vi "uv decode.vi"(8 "error in (no error)":errorcluster, 9 "para2":cluster{}, 10 "para1":cluster{}, 11 "para0":cluster{}) -> (0 "error out":errorcluster, 1 "function return":i32, 2 "para1 out":cluster{}, 3 "para0 out":cluster{})   [LabVIEW 2018]
doc: "LIBTIFF_DLL_IMPEXP int uv_decode(double*, double*, int);\nextern int uv_decode(double*, double*, int);"
uses:
  libtiff3.dll
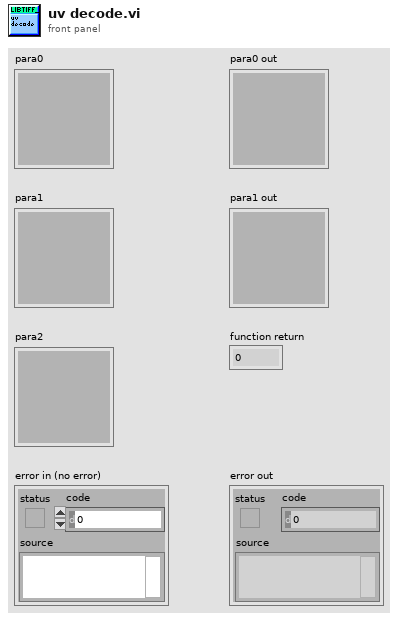
[diagram p1: front panel]
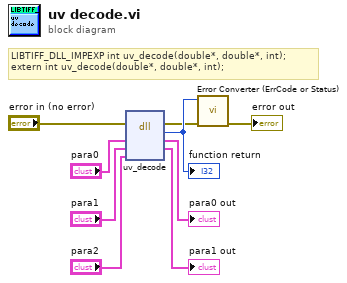
[diagram p0: block diagram]
diagram:
  # "LIBTIFF_DLL_IMPEXP\tint uv_decode(double*, double*, int);\nextern\tint uv_decode(double*, double*, int);"
  n1 = dll-call lib="C:/Users/johan/Downloads/LabVIEW software/LabVIEW software/IX-81 Software/lib/tiff/LibTiffLabview/libtiff3.*" fn="uv_decode"(error in="error in (no error)", "para0"="para0", "para1"="para1", "para2"="para2") -> (error out=w2:errorcluster, w9:i32, "para0"=→"para0 out":cluster{}, "para1"=→"para1 out":cluster{})  [unwired: 3 in, 1 out]
  "function return" <- w9
  n2 = call "Error Converter (ErrCode or Status).vi"("error in (no error)"=w2, "error code"=w9) -> ("error out"=→"error out":errorcluster)  [unwired: 9 in]
